vi "运维调试_CODMn.vi"() -> ()   [LabVIEW 2016, in "斯坦道CODMn新电路板.lvlib"]
uses:
  <vilib>/Utility/miscctls.llb/LVPointTypeDef.ctl
  <vilib>/Waveform/WDTFileIO.llb/Read Waveform from File.vi
  <vilib>/ptbypt/NI_PtbyPt.lvlib
panel:
  in  "告警代码":u16
  in  "周期设置":bool
  out "消解压力kPa":sgl format="%#.2f"
  out "权限等级":string
  out "总步数":i32
  out "滑动杆":u8(slide) caption="测试进度" scale=0.0..100.0
  in  "参数查询":bool
  in  "仪器校准":bool
  out "仪器版本号":string
  in  "试剂余量设置":bool
  out "试剂余量显示":sgl[][](graph)
  in  "公式切换阈值滴定数(0~9999)":dbl
  out "X0":u16
  in  "平台反控标样校准":enum16{"标液1", "标液2", "标液3"}(ring)
  in  "平台反控校准量程":enum16{"低量程1", "低量程2", "高量程1", "高量程2"}(ring)
  out "注射泵保温温度":sgl format="%#.2f"
  in  "历史波形 2":bool
  in  "返回 3":bool
  out "时间-温度":u16[](array[numeric]) caption="数组"
  out "温度波形时间":timestamp
  out "ORP滴定曲线 2":u16[](graph)
  in  "历史波形":bool
  in  "返回 2":bool
  out "滴定数-ORP值":u16[](array[numeric]) caption="数组"
  out "波形时间":timestamp
  out "ORP滴定曲线":u16[](graph)
  in  "滴定曲线":bool
  out "终点滴定数":sgl format="%#.2f"
  out "单位:":T1(ring)
  out "运行状态":T2 {"数据时间:" format="%<%y/%m/%d %H:%M:%S>T"; "仪器时间:" format="%<%y/%m/%d %H:%M:%S>T"}
  out "模块版本号":string
  out "当前步骤剩余时间":sgl format="%#.2f"
  out "加热实时温度":sgl format="%#.2f"
  out "ORP值/光值":sgl format="%#.2f"
  in  "布尔":bool
  in  "流程固件":bool
  in  "公式单个写入":bool
  in  "流程路径":path=path "C:/Users/STD/Documents/斯坦道流程文件/流程.xml"
  out "字符串":string
  out "运行时间":sgl format="%#.2f"
  out "环境湿度":sgl format="%#.2g"
  out "环境温度":sgl format="%#.2g"
  in  "数组":string[](array[string])
  in  "量程切换阈值写入":bool
  in  "量程切换阈值读取":bool
  in  "参数下拉列表":enum16{"CODMn"}(ring)
  in  "量程下拉列表":enum16{"低量程1", "低量程2", "高量程1", "高量程2"}(ring)
  in  "测量模式下拉列表":T3(ring)=enum."水样测量"
  in  "公式":cluster{"X^2":dbl, "X":dbl, "b":dbl}
  in  "写公式":bool
  in  "读公式":bool
  in  "返回":bool
  in  "设置":bool
  out "集成报警信息":string
  in  "停止":bool
  in  "手动启动":bool
  in  "单步测试":bool
  out "当前滴定数":sgl format="%#.2f"
  out "K":sgl format="%#.2f"
  out "B":sgl format="%#.2f"
  out "A":sgl format="%#.2f"
  out "多列列表框":i32(listbox)
  # "."
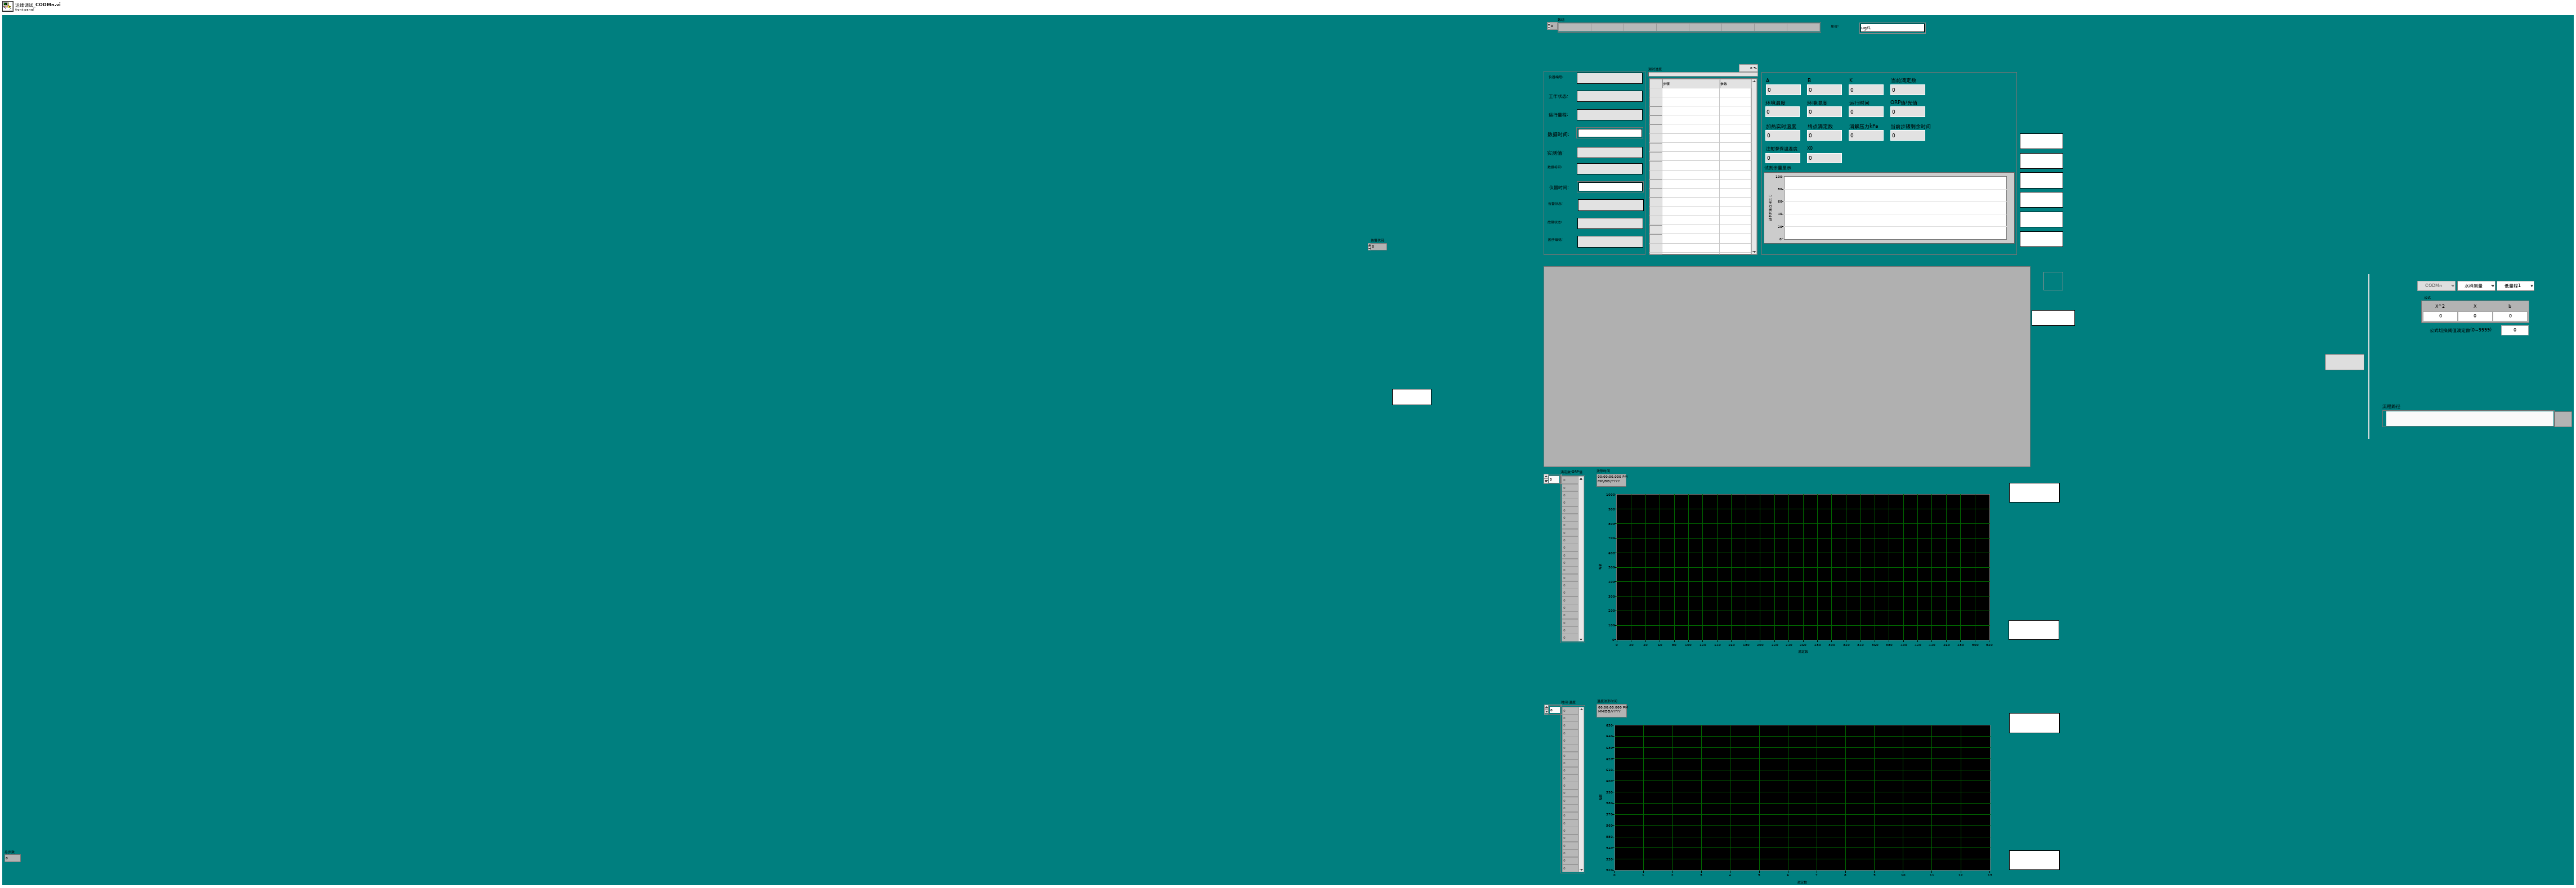
[diagram p1: front panel]
types:
  T1 = enum16{"ug/L", "mg/L", "ppm", "mg/m3", "cm", "ppb", "ug/m3", "%", "nmol/mol", "umol/mol", "MPN/L", "MPN/100ml", "ng/m3", "NTU", "无量纲", "ms/cm", "us/cm", "℃", "mV", "万个/L"}
  T2 = cluster{"仪器编号:":string, "工作状态:":string, "运行量程: ":string, "数据时间:":timestamp, "实测值:":string, "数据标识: ":string, "仪器时间:":timestamp, "告警状态: ":string, "故障状态:  ":string, "因子编码:":string}
  T3 = enum16{"", "水样测量", "标样核查", "零点核查", "跨度核查", "空白测试", "平行样测试", "加标回收"}
  T4 = cluster{"Major":u16, "Minor":u16, "Fix":u16, "Build":u16}
  T5 = cluster{"测量量程":sgl, "测量检出限":sgl, "测量精度":sgl, "测量间隔":sgl, "消解温度":sgl, "消解时长":sgl, "三项式系数":sgl, "二次多项式系数":sgl, "曲线斜率":sgl, "曲线截距":sgl, "线性相关系数":sgl, "空白校准时间":timestamp, "标样校准时间":timestamp, "测量信号值":sgl, "稀释倍数":sgl, "量程系数":sgl}
  T6 = typedef "LVPointTypeDef.ctl" = cluster{"Horizontal":i16, "Vertical":i16}
  T7 = cluster{"因子编码":u32, "单位":u16, "标样参考值":sgl, "水样数据时间":timestamp, "水样实测值":sgl, "水样数据标识":string, "标样数据时间":timestamp, "标样实测值":sgl, "标样数据标识":string, "空白数据时间":timestamp, "空白实测值":sgl, "空白数据标识":string, "零点核查数据时间":timestamp, "零点核查实测值":sgl, "零点核查数据标识":string, "跨度核查数据时间":timestamp, "跨度核查实测值":sgl, "跨度核查数据标识":string, "加标回收数据时间":timestamp, "加标回收实测值":sgl, "加标回收数据标识":string, "平行样数据时间":timestamp, "平行样实测值":sgl, "平行样数据标识":string, "F0":sgl, "F1":sgl, "F2":sgl, "F3":sgl, "F4":sgl, "F5":sgl, "F6":sgl, "F7":sgl, "温度":sgl, "湿度":sgl, "X值":sgl, "fidrange":u16}
  T8 = cluster{"系统时间":timestamp, "工作状态":u16, "测量模式":enum16{"待机", "连续模式", "周期模式", "定点模式", "受控模式", "手动模式"}, "告警代码":u16, "故障代码":u16, "日志代码":u16, "软件版本":u16, "A":sgl, "B":sgl, "K":sgl, "当前滴定数":sgl, "T":sgl, "H":sgl, "id":u16, "flowid":u16, "量程":u16, "加热实时温度":sgl, "当前ORP值":sgl, "运行时间":sgl, "当前步骤剩余时间":sgl, "结束滴定数":sgl, "注射泵保温温度":sgl, "匹配滴定数X0":u16, "X^2":sgl, "X":sgl, "B 2":sgl, "光值1":sgl, "光值2":sgl, "光值3":sgl, "光值4":sgl, "光值5":sgl, "光值6":sgl, "光值7":sgl, "光值8":sgl}
  T9 = typedef "Alarm interface.lvlib/报警短信语音交互.ctl" = cluster{"参数":string, "元器件":string, "故障现象":string, "code":string, "platform_alarm_code":string, "solutionList":cluster{"reason":string, "solution":string}[], "是否上报":string}
  T10 = enum8{"Enabled", "Disabled", "Disabled and Grayed Out"}
  T11 = enum16{"空闲", "水样测试", "标样核查", "零点核查", "跨度核查", "空白测试", "平行样测试", "加标回收", "空白校准", "标样校准", "初始化（清洗）"}
  T12 = typedef "TimingControl.lvlib/TimingControl.lvclass/国标控制命令.ctl" = enum16{"启动测量", "标样核查", "零点核查", "跨度核查", "空白测试", "平行样测试", "加标回收", "空白校准", "标样校准", "初始化（清洗）", "停止测试", "仪器重启", "校时", "模式设置", "测量间隔设置"}
  T13 = typedef "TimingControl.lvlib/TimingControl.lvclass/测量参数.ctl" = u16
  T14 = cluster{"时间标识":timestamp, "设备":string, "日志信息":string, "流程参数":string}
  T15 = typedef "LVRowAndColumnUnsignedTypeDef.ctl" = cluster{"Row":u32, "Column":u32}
  T16 = enum32{"Bad", "Idle", "Run top level", "Running"}
  T17 = cluster{"站号":u16, "量程切换":enum32{"H", "L", "AUTO"}, "控制命令":u16, "模式设置":enum16{"待机", "连续模式", "周期模式", "定点模式", "受控模式", "手动模式"}, "测量间隔":u16}
  T18 = cluster{"测量量程":dbl, "测量精度":dbl, "测量间隔":dbl, "消解温度":dbl, "消解时长":dbl, "空白校准时间":timestamp, "曲线截距":dbl, "曲线斜率":dbl, "测量检出限":dbl, "测量信号值":dbl, "线性相关系数":dbl, "二次多项式系数":dbl, "标样校准时间":timestamp, "稀释倍数":dbl, "三项式系数":dbl, "空白标定系数":dbl, "量程系数":dbl, "F0/ORPA":dbl, "F1/ORPB":dbl, "F2/ORPK":dbl, "F3":dbl, "F4":dbl, "F5":dbl, "F6":dbl, "F7":dbl, "X0/滴定数":dbl, "量程":dbl}
  T19 = cluster{"跨度值":dbl, "零点标准液浓度":dbl, "跨度标准液浓度":dbl, "标准液标准浓度":dbl, "零点标准液偏差":dbl, "跨度标准液偏差":dbl, "标准液标准偏差":dbl}
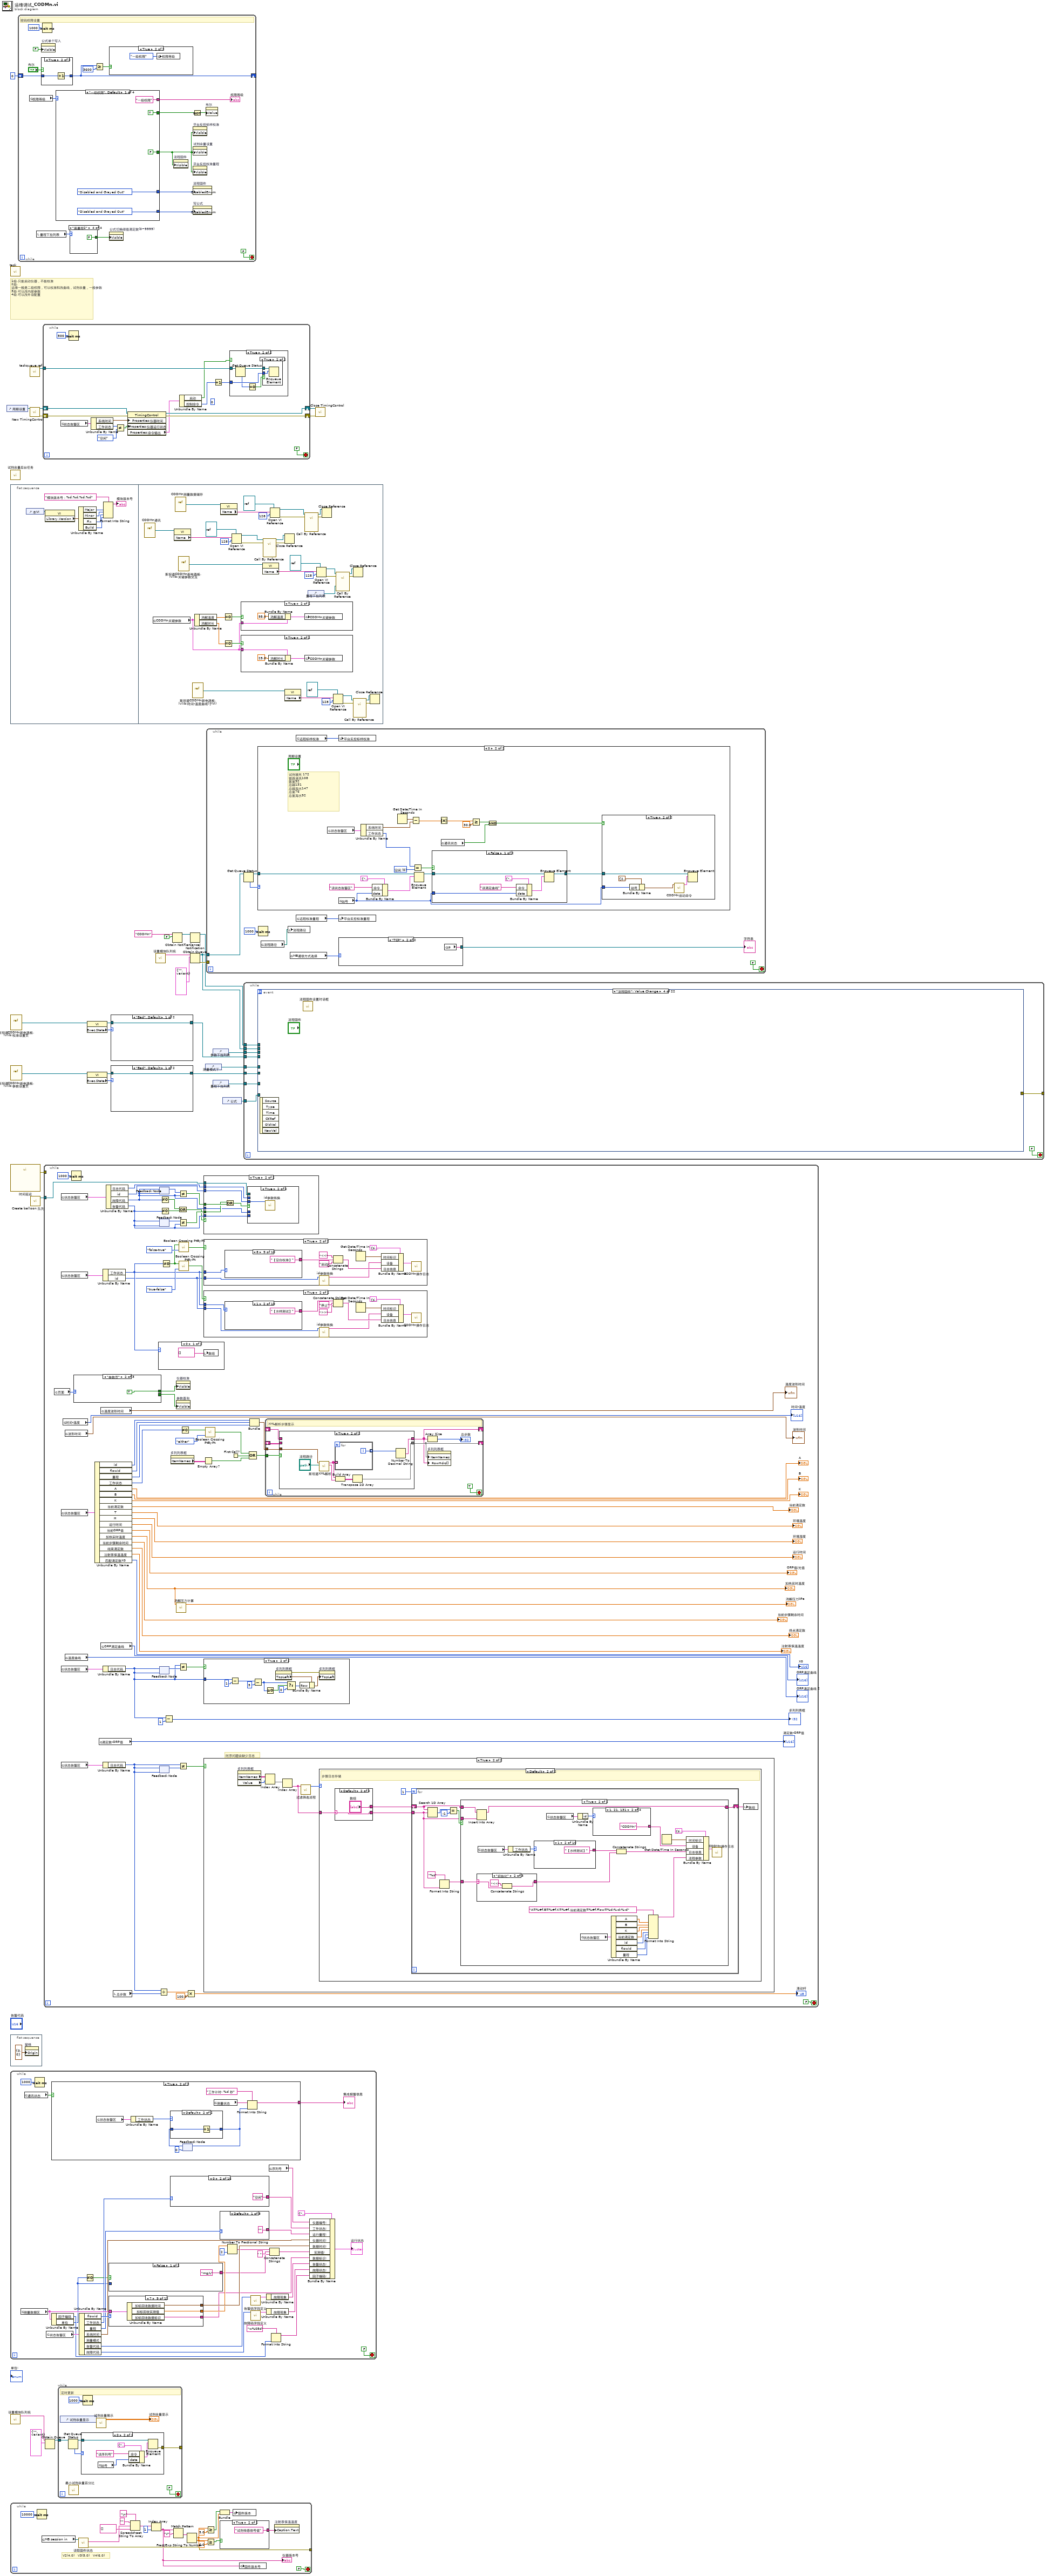
[diagram p0: block diagram]
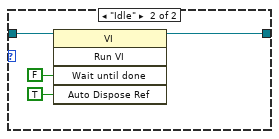
[diagram p2: hidden frame]
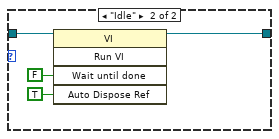
[diagram p3: hidden frame]
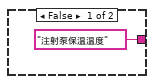
[diagram p4: hidden frame]
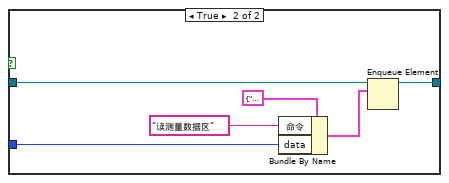
[diagram p7: hidden frame]
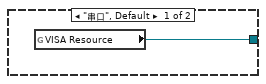
[diagram p9: hidden frame]
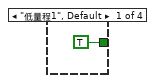
[diagram p12: hidden frame]
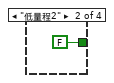
[diagram p13: hidden frame]
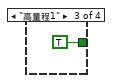
[diagram p14: hidden frame]
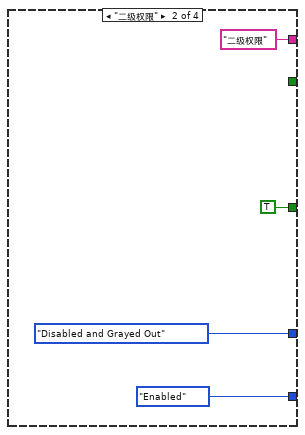
[diagram p15: hidden frame]
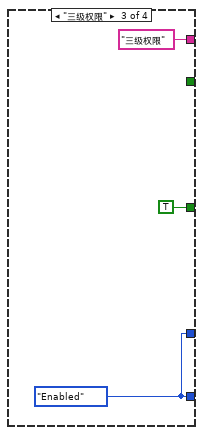
[diagram p16: hidden frame]
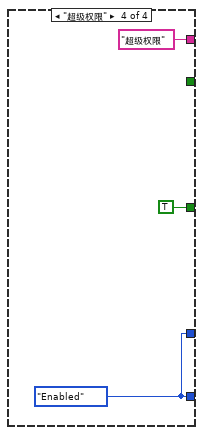
[diagram p17: hidden frame]
diagram:
  # "1级.只能启动仪器，不能校准\n2级.运维一般是二级权限，可以校准和改曲线，试剂余量，一般参数\n3级.可以改内部参数\n4级.可以改外设配置"
  n1 = control-ref of="周期设置"() -> (w5:refnum<vi>)
  n2 = call "task.vi"() -> ()  [unwired: 12 in]
  n3 = call "试剂余量后台任务.vi"() -> ()  [unwired: 12 in]
  n4 = flat-sequence {
    frame #0 {
      n5 = control-ref of="本VI"() -> (w40:refnum<vi>)
      n6 = property class="VI"(reference=w40) -> ("Library.Version"=w39:T4)  [unwired: 1 in, 2 out]
      n7 = Unbundle By Name(w39) -> ("Major"=w37:u16, "Minor"=w36:u16, "Fix"=w35:u16, "Build"=w34:u16)
      n8 = Format Into String(format string="模块版本号：%d.%d.%d.%d" ("格式字符串"), w37, w36, w35, w34) -> (resulting string=→"模块版本号":string)  [unwired: 2 in, 1 out]
    }
    frame #1 {
      n9 = vi-ref "CODMn通讯.vi"() -> (w54:refnum<vi>)
      n10 = global read "CODMn断电保存全局变量.vi" "CODMn关键参数"() -> (w41:T5)
      n11 = property class="VI"(reference=w54) -> ("Name"=w53:string)  [unwired: 1 in, 2 out]
      n12 = vi-ref "CODMn测量数据储存.vi"() -> (w78:refnum<vi>)
      n13 = vi-ref "斯坦道CODMn新电路板.lvlib:关键参数交互.vi"() -> (w64:refnum<vi>)
      n14 = vi-ref "斯坦道CODMn新电路板.lvlib:时间-温度曲线(子VI).vi"() -> (w56:refnum<vi>)
      n15 = Unbundle By Name(w41) -> ("消解温度"=w45:sgl, "消解时长"=w42:sgl)
      n16 = property class="VI"(reference=w78) -> ("Name"=w71:string)  [unwired: 1 in, 2 out]
      n17 = Equal To 0?(x=w45) -> (x = 0?=w44:bool)
      n18 = Equal To 0?(x=w42) -> (x = 0?=w43:bool)
      n19 = Open VI Reference(type specifier VI Refnum (for type only)=refnum<vi> refnum, vi path=w53, options=128 ("选项")) -> (vi reference=w51:refnum<vi>, error out=w49:errorcluster)  [unwired: 3 in]
      n20 = case shown="True" w44 {
        tunnel: w41 -> [_ w84]
        frame False {
        }
        frame True {
          n21 = Bundle By Name(cluster=w84, "消解温度"=sgl 95.0) -> (w83:T5)
          n22 = global write "CODMn断电保存全局变量.vi" "CODMn关键参数"(w83) -> ()
        }
      }
      n23 = case shown="True" w43 {
        tunnel: w41 -> [_ w81]
        frame False {
        }
        frame True {
          n24 = Bundle By Name(cluster=w81, "消解时长"=sgl 25.0) -> (w80:T5)
          n25 = global write "CODMn断电保存全局变量.vi" "CODMn关键参数"(w80) -> ()
        }
      }
      n26 = property class="VI"(reference=w64) -> ("Name"=w70:string)  [unwired: 1 in, 2 out]
      n27 = call-by-ref "?"(reference=w51, error in=w49) -> (reference out=w47:refnum<vi>, error out=w48:errorcluster)  [unwired: 12 in]
      n28 = Open VI Reference(type specifier VI Refnum (for type only)=refnum<vi> refnum, vi path=w71, options=128 ("选项")) -> (vi reference=w73:refnum<vi>, error out=w75:errorcluster)  [unwired: 3 in]
      n29 = Close Reference(reference=w47, error in (no error)=w48) -> ()  [unwired: 1 out]
      n30 = property class="VI"(reference=w56) -> ("Name"=w62:string)  [unwired: 1 in, 2 out]
      n31 = call-by-ref "?"(reference=w73, error in=w75) -> (reference out=w77:refnum<vi>, error out=w76:errorcluster)  [unwired: 12 in]
      n32 = control-ref of="量程下拉列表"() -> (w46:refnum<vi>)
      n33 = Open VI Reference(type specifier VI Refnum (for type only)=refnum<vi> refnum, vi path=w70, options=128 ("选项")) -> (vi reference=w68:refnum<vi>, error out=w67:errorcluster)  [unwired: 3 in]
      n34 = Close Reference(reference=w77, error in (no error)=w76) -> ()  [unwired: 1 out]
      n35 = Open VI Reference(type specifier VI Refnum (for type only)=refnum<vi> refnum, vi path=w62, options=128 ("选项")) -> (vi reference=w60:refnum<vi>, error out=w59:errorcluster)  [unwired: 3 in]
      n36 = call-by-ref "?"(reference=w68, error in=w67, "量程下拉列表"=w46) -> (reference out=w65:refnum<vi>, error out=w66:errorcluster)  [unwired: 11 in]
      n37 = Close Reference(reference=w65, error in (no error)=w66) -> ()  [unwired: 1 out]
      n38 = call-by-ref "?"(reference=w60, error in=w59) -> (reference out=w57:refnum<vi>, error out=w58:errorcluster)  [unwired: 12 in]
      n39 = Close Reference(reference=w57, error in (no error)=w58) -> ()  [unwired: 1 out]
    }
  }
  n40 = vi-ref "斯坦道CODMn新电路板.lvlib:校准设置页.vi"() -> (w16:refnum<vi>)
  n41 = vi-ref "斯坦道CODMn新电路板.lvlib:参数设置页.vi"() -> (w13:refnum<vi>)
  n42 = call "时间延迟"() -> ("error out"=w26:errorcluster)  [unwired: 11 in]
  n43 = flat-sequence {
    frame #0 {
      n44 = property on="窗格" class="Pane"("Origin"=T6 {"Horizontal"=0, "Vertical"=0} ("原点")) -> ()  [unwired: 2 in, 2 out]
    }
  }
  n45 = while {
    stop <- FALSE stop-if-true
    n46 = global read "VARCODMn全局变量.vi" "测量数据区"() -> (w113:T7)
    n47 = global read "VARCODMn全局变量.vi" "通讯状态"() -> (w117:bool)
    n48 = Wait (ms)(milliseconds to wait=u32 1000 ("等待时间（毫秒）")) -> ()  [unwired: 1 out]
    n49 = global read "VARCODMn全局变量.vi" "状态告警区"() -> (w115:T8)
    n50 = case shown="True" w117 {
      tunnel: ["通讯异常" ("集成报警信息") w195] -> w116
      frame False {
      }
      frame True {
        n51 = global read "VARCODMn全局变量.vi" "状态告警区"() -> (w201:T8)
        n52 = Unbundle By Name(w201) -> ("工作状态"=w200:u16)
        n53 = feedback #1(0) -> (w198:i32)
        n54 = case shown="Default" w200 {
          tunnel: w198 -> [_ w203]
          tunnel: [_ w202] -> w196
          frame 0 {
          }
          frame Default {
            n55 = Increment(x=w203) -> (x+1=w202:i32)
          }
        }
        n56 = feedback-in #1(w196) -> ()
        n57 = global read "VARCODMn全局变量.vi" "测量状态"() -> (w194:string)
        n58 = Format Into String(format string="工作计时: %d 秒" ("格式字符串"), initial string=w194, w196) -> (resulting string=w195:string)  [unwired: 1 in, 1 out]
      }
    }
    "集成报警信息" <- w116
    n59 = Unbundle By Name(w113) -> ("因子编码"=w93:u32, "单位"=w90:u16)
    n60 = Unbundle By Name(w115) -> ("flowid"=w114:u16, "工作状态"=w111:u16, "量程"=w109:u16, "系统时间"=w107:timestamp, "告警代码"=w97:u16, "故障代码"=w96:u16)  [unwired: 1 out]
    n61 = Not Equal To 0?(x=w90) -> (x != 0?=w91:bool)
    n62 = case shown="False" w91 {
      tunnel: ["mg/L" ("RingText.Text") w122] -> w95
      tunnel: w90 -> [_ w121]
      frame False {
      }
      frame True {
        n63 = property on="单位:" class="Enum (strict)"("Value"=w121) -> (error out=w123:errorcluster)  [unwired: 2 in, 1 out]
        n64 = property on="单位:" class="Enum (strict)"(error in=w123) -> ("RingText.Text"=w122:string)  [unwired: 1 in, 2 out]
      }
    }
    n65 = case shown="7" w114 {
      selector: w114 -> [w146 _ _ _ _ _ _ _ _ _ _ _]
      tunnel: [_ w152 w156 w160 w164 w168 w172 w176 w180 w183 w187 w192] -> w104
      tunnel: [_ w150 w155 w159 w163 w167 w171 w174 w179 w182 w186 w191] -> w99
      tunnel: [_ w149 w154 w158 w162 w166 w170 w173 w178 w181 w185 w190] -> w98
      tunnel: w113 -> [_ w151 w153 w157 w161 w165 w169 w175 w177 w184 w188 w189]
      frame Default {
        n66 = Format Into String(format string="%d" ("格式字符串"), initial string="未知" ("工作状态"), w146) -> ()  [unwired: 1 in, 2 out]
      }
      frame 0 {
        n67 = Unbundle By Name(w151) -> ("水样数据时间"=w152:timestamp, "水样实测值"=w150:sgl, "水样数据标识"=w149:string)
      }
      frame 1 {
        n68 = Unbundle By Name(w153) -> ("水样数据时间"=w156:timestamp, "水样实测值"=w155:sgl, "水样数据标识"=w154:string)
      }
      frame 2 {
        n69 = Unbundle By Name(w157) -> ("标样数据时间"=w160:timestamp, "标样实测值"=w159:sgl, "标样数据标识"=w158:string)
      }
      frame 3 {
        n70 = Unbundle By Name(w161) -> ("零点核查数据时间"=w164:timestamp, "零点核查实测值"=w163:sgl, "零点核查数据标识"=w162:string)
      }
      frame 4 {
        n71 = Unbundle By Name(w165) -> ("跨度核查数据时间"=w168:timestamp, "跨度核查实测值"=w167:sgl, "跨度核查数据标识"=w166:string)
      }
      frame 5 {
        n72 = Unbundle By Name(w169) -> ("空白数据时间"=w172:timestamp, "空白实测值"=w171:sgl, "空白数据标识"=w170:string)
      }
      frame 6 {
        n73 = Unbundle By Name(w175) -> ("平行样数据时间"=w176:timestamp, "平行样实测值"=w174:sgl, "平行样数据标识"=w173:string)
      }
      frame 7 {
        n74 = Unbundle By Name(w177) -> ("加标回收数据时间"=w180:timestamp, "加标回收实测值"=w179:sgl, "加标回收数据标识"=w178:string)
      }
      frame 8 {
        n75 = Unbundle By Name(w184) -> ("空白数据时间"=w183:timestamp, "空白实测值"=w182:sgl, "空白数据标识"=w181:string)
      }
      frame 9 {
        n76 = Unbundle By Name(w188) -> ("标样数据时间"=w187:timestamp, "标样实测值"=w186:sgl, "标样数据标识"=w185:string)
      }
      frame 10 {
        n77 = Unbundle By Name(w189) -> ("水样数据时间"=w192:timestamp, "水样实测值"=w191:sgl, "水样数据标识"=w190:string)
      }
    }
    n78 = case shown="0" w111 {
      selector: w111 -> [w127 _ _ _ _ _ _ _ _ _ _ _ _ _ _ _]
      tunnel: [w128 "空闲" ("工作状态") "水样测量" ("工作状态") "标样核查" ("工作状态") "零点核查" ("工作状态") "跨度核查" ("工作状态") "空白测试" ("工作状态") "平行样测试" ("工作状态") "加标回收" ("工作状态") "空白校准" ("工作状态") "标样校准" ("工作状态") "初始化" ("工作状态") "调试" ("工作状态") "填充管路" ("工作状态") "清洗管路" ("工作状态") "清洗反应杯" ("工作状态")] -> w110
      frame Default {
        n79 = Format Into String(format string="%d" ("格式字符串"), initial string="未知" ("工作状态"), w127) -> (resulting string=w128:string)  [unwired: 1 in, 1 out]
      }
      frame 0 {
      }
      frame 1 {
      }
      frame 2 {
      }
      frame 3 {
      }
      frame 4 {
      }
      frame 5 {
      }
      frame 6 {
      }
      frame 7 {
      }
      frame 8 {
      }
      frame 9 {
      }
      frame 10 {
      }
      frame 22 {
      }
      frame 30 {
      }
      frame 31 {
      }
      frame 32 {
      }
    }
    n80 = case shown="Default" w109 {
      tunnel: ["" ("字符串") "低量程" ("字符串") "高量程" ("字符串")] -> w108
      frame Default {
      }
      frame 0 {
      }
      frame 1 {
      }
    }
    n81 = Number To Fractional String(number=w99, precision (6)=i16 2 ("精度(6)")) -> (F-format string=w102:string)  [unwired: 2 in]
    n82 = call "告警码字段定义.vi"("告警代码"=w97) -> ("data"=w89:T9)  [unwired: 10 in]
    n83 = call "故障码字段定义.vi"("故障代码"=w96) -> ("data"=w88:T9)  [unwired: 10 in]
    n84 = Unbundle By Name(w89) -> ("故障现象"=w86:string)
    n85 = Unbundle By Name(w88) -> ("故障现象"=w87:string)
    n86 = global read "VARCODMn全局变量.vi" "序列号"() -> (w112:string)
    n87 = Concatenate Strings(w102, " " ("字符串"), w95) -> (w100:string)
    n88 = Format Into String(format string="w%05d" ("格式字符串"), w93) -> (resulting string=w92:string)  [unwired: 2 in, 1 out]
    n89 = Bundle By Name(cluster=T2 {"仪器编号:"="", "工作状态:"="", "运行量程: "="", "数据时间:"=timestamp(0 s since 1904-01-01), "实测值:"="", "数据标识: "="", "仪器时间:"=timestamp(0 s since 1904-01-01), "告警状态: "="", "故障状态:  "="", "因子编码:"=""} ("运行状态"), "仪器编号:"=w112, "工作状态:"=w110, "运行量程:"=w108, "仪器时间:"=w107, "数据时间:"=w104, "实测值:"=w100, "数据标识:"=w98, "告警状态:"=w86, "故障状态:"=w87, "因子编码:"=w92) -> (→"运行状态":T2)
  }
  n90 = call "设置模块队列名.vi"() -> ("Msg"=w6:string)  [unwired: 11 in]
  n91 = while {
    tunnel: [w220] -> _
    stop <- FALSE stop-if-true
    # "V2(4.0)   V3(5.0)   V4(6.0)"
    n92 = Wait (ms)(milliseconds to wait=u32 10000 ("等待时间（毫秒）")) -> ()  [unwired: 1 out]
    n93 = global read "VARCODMn全局变量.vi" "MB session in"() -> (w221:refnum<class "MB_Master.lvclass">)
    n94 = call "读取固件状态.vi"("MB session in"=w221) -> ("error out"=w220:errorcluster, "结果字符串"=w216:string)  [unwired: 8 in, 1 out]
    n95 = Spreadsheet String To Array(delimiter (Tab)="\n" ("分隔符(Tab)"), format string="" ("格式字符串"), spreadsheet string=w216, array type (2D Dbl)=string[] []) -> (array=w215:string[])
    n96 = Index Array(array=w215, index=1 ("索引")) -> (element=w204:string)
    "仪器版本号" <- w204
    n97 = Match Pattern(string=w204, regular expression="V" ("正则表达式")) -> (after substring=w212:string)  [unwired: 1 in, 3 out]
    n98 = Fract/Exp String To Number(string=w212) -> (number=w206:dbl)  [unwired: 3 in, 1 out]
    n99 = Greater Or Equal?(x=w206, y=5.0) -> (x >= y?=w207:bool)
    n100 = Greater Or Equal?(x=w206, y=6.0) -> (x >= y?=w209:bool)
    n101 = Bundle(w207, w206) -> (w205:cluster{bool, dbl})  [unwired: 1 in]
    n102 = case shown="True" w209 {
      tunnel: ["注射泵保温温度" "试剂传感信号值"] -> w208
      frame False {
      }
      frame True {
      }
    }
    n103 = global write "VARCODMn全局变量.vi" "固件版本"(w205) -> ()
    n104 = global write "VARCODMn全局变量.vi" "固件版本号"(w204) -> ()
    n105 = property on="注射泵保温温度" class="DigNum (strict)"("Caption.Text"=w208) -> ()  [unwired: 2 in, 2 out]
  }
  n106 = while {
    shift-right: [w239] -> _
    shift-left: u32 0 ("等待时间（毫秒）") -> [w240]
    stop <- FALSE stop-if-true
    # "密码权限设置"
    n107 = global read "VARCODMn全局变量.vi" "权限等级"() -> (w231:enum16{"一级权限", "二级权限", "三级权限", "超级权限"})
    n108 = local read "量程下拉列表"() -> (w233:enum16{"低量程1", "低量程2", "高量程1", "高量程2"})
    n109 = property on="公式单个写入" class="Bool"("Visible"=FALSE ("可见")) -> ()  [unwired: 2 in, 2 out]
    n110 = case shown="True" "布尔" {
      tunnel: w240 -> [_ w264]
      tunnel: [_ w263] -> w239
      frame False {
      }
      frame True {
        n111 = Increment(x=w264) -> (x+1=w263:u32)
      }
    }
    n112 = Wait (ms)(milliseconds to wait=u32 1000 ("等待时间（毫秒）")) -> ()  [unwired: 1 out]
    n113 = case shown="\"一级权限\", Default" w231 {
      tunnel: [T10."Disabled and Grayed Out" ("f") T10."Enabled" ("禁用") w258 w261] -> w234
      tunnel: [T10."Disabled and Grayed Out" ("f") T10."Disabled and Grayed Out" ("f") w258 w261] -> w235
      tunnel: [FALSE ("可见") TRUE ("可见") TRUE ("可见") TRUE ("可见")] -> w230
      tunnel: ["一级权限" "二级权限" "三级权限" "超级权限"] -> w229
      tunnel: [TRUE _ _ _] -> w228
      frame "一级权限", Default {
      }
      frame "二级权限" {
      }
      frame "三级权限" {
        w258 = T10."Enabled" ("禁用")
      }
      frame "超级权限" {
        w261 = T10."Enabled" ("禁用")
      }
    }
    "权限等级" <- w229
    n114 = case shown="\"高量程2\"" w233 {
      tunnel: [TRUE ("可见") FALSE ("可见") TRUE ("可见") FALSE ("可见")] -> w232
      frame "低量程1", Default {
      }
      frame "低量程2" {
      }
      frame "高量程1" {
      }
      frame "高量程2" {
      }
    }
    n115 = Greater Or Equal?(x=w239, y=u32 3600) -> (x >= y?=w237:bool)
    n116 = case shown="True" w237 {
      frame False {
      }
      frame True {
        n117 = global write "VARCODMn全局变量.vi" "权限等级"(enum16{"一级权限", "二级权限", "三级权限", "超级权限"}."一级权限" ("权限等级")) -> ()
      }
    }
    n118 = property on="公式切换阈值滴定数(0~9999)" class="DigNum (strict)"("Visible"=w232) -> ()  [unwired: 2 in, 2 out]
    n119 = property on="流程固件" class="Bool"("Visible"=w230) -> ()  [unwired: 2 in, 2 out]
    n120 = Not(x=w228) -> (.not. x?=w226:bool)
    n121 = property on="平台反控标样校准" class="Enum (strict)"("Visible"=w230) -> ()  [unwired: 2 in, 2 out]
    n122 = property on="试剂余量设置" class="Bool"("Visible"=w230) -> ()  [unwired: 2 in, 2 out]
    n123 = property on="平台反控校准量程" class="Enum (strict)"("Visible"=w230) -> ()  [unwired: 2 in, 2 out]
    n124 = property on="流程固件" class="Bool"("DisabledEnum"=w235) -> ()  [unwired: 2 in, 2 out]
    n125 = property on="写公式" class="Bool"("DisabledEnum"=w234) -> ()  [unwired: 2 in, 2 out]
    n126 = property on="布尔" class="Bool (strict)"("Value"=w226) -> ()  [unwired: 2 in, 2 out]
  }
  n127 = call "taskqueue ref.vi"() -> ("队列输出"=w8:refnum<queue>)  [unwired: 10 in, 1 out]
  n128 = call "New TimingControl.vi"("Reference"=w5) -> ("error out"=w3:errorcluster, "TimingControl out"=w4:refnum<class "TimingControl.lvclass">)  [unwired: 9 in]
  n129 = call "Create balloon 队列.vi"() -> ("队列输出"=w19:refnum<queue>)  [unwired: 11 in]
  n130 = while {
    tunnel: w8 -> [w276]
    shift-right: [w272] -> w2
    shift-left: w4 -> [w274]
    shift-right: [w271] -> w1
    shift-left: w3 -> [w273]
    stop <- FALSE stop-if-true
    (unwired) u32 0 ("f")
    n131 = global read "VARCODMn全局变量.vi" "状态告警区"() -> (w278:T8)
    n132 = Wait (ms)(milliseconds to wait=u32 500 ("等待时间（毫秒）")) -> ()  [unwired: 1 out]
    n133 = Unbundle By Name(w278) -> ("系统时间"=w269:timestamp, "工作状态"=w275:u16)
    n134 = Not Equal?(x=w275, y=T11."空闲") -> (x != y?=w268:bool)
    n135 = property class="TimingControl"(reference=w274, error in=w273, "Properties:仪器时间"=w269, "Properties:仪器运行状态"=w268) -> (reference out=w272:refnum<class "TimingControl.lvclass">, error out=w271:errorcluster, "Properties:命令输出"=w270:cluster{"启动":bool, "控制命令":T12, "测量参数":T13})
    n136 = Unbundle By Name(w270) -> ("启动"=w265:bool, "控制命令"=w267:T12)
    n137 = Increment(x=w267) -> (x+1=w266:T12)
    n138 = case shown="True" w265 {
      tunnel: w276 -> [_ w285]
      tunnel: w266 -> [_ w284]
      frame False {
      }
      frame True {
        n139 = Get Queue Status(queue=w285) -> (queue out=w283:refnum<queue>, # elements in queue=w282:i32)  [unwired: 2 in, 6 out]
        n140 = Equal To 0?(x=w282) -> (x = 0?=w281:bool)
        n141 = case shown="True" w281 {
          tunnel: w284 -> [_ w287]
          tunnel: w283 -> [_ w286]
          frame False {
          }
          frame True {
            n142 = Enqueue Element(queue=w286, element=w287) -> ()  [unwired: 2 in, 3 out]
          }
        }
      }
    }
  }
  n143 = while {
    tunnel: w26 -> [_]
    tunnel: w19 -> [w316]
    stop <- FALSE stop-if-true
    # "时序问题会缺少日志"
    n144 = global read "VARCODMn全局变量.vi" "页面"() -> (w293:enum16{"主页", "参数页", "校准页"})
    n145 = global read "VARCODMn全局变量.vi" "状态告警区"() -> (w344:T8)
    n146 = global read "VARCODMn全局变量.vi" "状态告警区"() -> (w340:T8)
    n147 = global read "VARCODMn全局变量.vi" "状态告警区"() -> (w353:T8)
    n148 = global read "VARCODMn全局变量.vi" "状态告警区"() -> (w319:T8)
    n149 = global read "VARCODMn全局变量.vi" "状态告警区"() -> (w338:T8)
    n150 = global read "VARCODMn全局变量.vi" "时间-温度"() -> (→"时间-温度":u16[])
    n151 = global read "VARCODMn全局变量.vi" "波形时间"() -> (→"波形时间":timestamp)
    n152 = global read "VARCODMn全局变量.vi" "温度曲线"() -> (→"ORP滴定曲线 2":u16[])
    n153 = Wait (ms)(milliseconds to wait=u32 1000 ("等待时间（毫秒）")) -> ()  [unwired: 1 out]
    n154 = case shown="\"参数页\"" w293 {
      tunnel: [_ _ TRUE ("可见")] -> w292
      tunnel: [_ TRUE ("可见") _] -> w291
      frame "主页", Default {
      }
      frame "参数页" {
      }
      frame "校准页" {
      }
    }
    n155 = Unbundle By Name(w353) -> ("id"=w350:u16, "flowid"=w352:u16, "量程"=w351:u16, "工作状态"=w330:u16, "A"=→"A":sgl, "B"=→"B":sgl, "K"=→"K":sgl, "当前滴定数"=→"当前滴定数":sgl, "T"=→"环境温度":sgl, "H"=→"环境湿度":sgl, "运行时间"=→"运行时间":sgl, "当前ORP值"=→"ORP值/光值":sgl, "加热实时温度"=w290:sgl, "当前步骤剩余时间"=→"当前步骤剩余时间":sgl, "结束滴定数"=→"终点滴定数":sgl, "注射泵保温温度"=→"注射泵保温温度":sgl, "匹配滴定数X0"=→"X0":u16)
    "加热实时温度" <- w290
    n156 = global read "VARCODMn全局变量.vi" "滴定数-ORP值"() -> (→"滴定数-ORP值":u16[])
    n157 = global read "VARCODMn全局变量.vi" "温度波形时间"() -> (→"温度波形时间":timestamp)
    n158 = global read "VARCODMn全局变量.vi" "ORP滴定曲线"() -> (→"ORP滴定曲线":u16[])
    n159 = Unbundle By Name(w340) -> ("工作状态"=w323:u16, "id"=w322:u16)
    n160 = Unbundle By Name(w319) -> ("日志代码"=w335:u16)
    n161 = Unbundle By Name(w338) -> ("日志代码"=w296:u16)
    n162 = Unbundle By Name(w344) -> ("日志代码"=w288:u16, "id"=w343:u16, "故障代码"=w302:u16, "告警代码"=w301:u16)
    n163 = local read "总步数"() -> (w295:i32)
    n164 = case shown="0" w323 {
      frame 0 {
        n165 = local write "数组"(string[] [] ("数组")) -> ()
      }
      frame 1, Default {
      }
    }
    n166 = Divide(x=w296, y=w295) -> (x/y=w298:dbl)
    n167 = feedback #2(w302) -> (w341:u16)
    n168 = feedback-in #2(w302) -> ()
    n169 = feedback #3(w301) -> (w318:u16)
    n170 = feedback-in #3(w301) -> ()
    n171 = feedback-in #4(w335) -> ()
    n172 = feedback #4(w335) -> (w358:u16)
    n173 = feedback #5(w296) -> (w339:u16)
    n174 = feedback-in #5(w296) -> ()
    n175 = Not Equal To 0?(x=w302) -> (x != 0?=w304:bool)
    n176 = Not Equal To 0?(x=w301) -> (x != 0?=w303:bool)
    n177 = Not Equal To 0?(x=w323) -> (x != 0?=w325:bool)
    n178 = Subtract(x=w335, y=1) -> (x-y=→"多列列表框":i32)
    n179 = property on="多列列表框" class="MCListbox (strict)"() -> ("ItemNames"=w314:string[][])  [unwired: 2 in, 2 out]
    n180 = property on="仪器校准" class="Bool"("Visible"=w291) -> ()  [unwired: 2 in, 2 out]
    n181 = property on="参数查询" class="Bool"("Visible"=w292) -> ()  [unwired: 2 in, 2 out]
    n182 = call "消解压力计算.vi"("当前消解温度"=w290) -> ("消解压力"=→"消解压力kPa":dbl)  [unwired: 10 in]
    n183 = Or(x=w304, y=w303) -> (x .or. y?=w300:bool)
    n184 = Not Equal?(x=w341, y=w302) -> (x != y?=w342:bool)
    n185 = Not Equal?(x=w318, y=w301) -> (x != y?=w317:bool)
    n186 = Not Equal?(x=w335, y=w358) -> (x != y?=w357:bool)
    n187 = Not Equal?(x=w296, y=w339) -> (x != y?=w337:bool)
    n188 = call <vilib>:"Boolean Crossing PtByPt.vi"("direction"=enum16{"either", "false-true", "true-false"}."false-true", "input"=w325) -> ("crossing"=w327:bool)  [unwired: 1 in]
    n189 = call <vilib>:"Boolean Crossing PtByPt.vi"("direction"=enum16{"either", "false-true", "true-false"}."true-false", "input"=w325) -> ("crossing"=w324:bool)  [unwired: 1 in]
    n190 = Not Equal To 0?(x=w330) -> (x != 0?=w355:bool)
    n191 = Multiply(x=w298, y=100.0) -> (x*y=→"滑动杆":dbl)
    n192 = case shown="True" w300 {
      tunnel: w343 -> [_ w476]
      tunnel: w342 -> [_ w475]
      tunnel: w317 -> [_ w473]
      tunnel: w301 -> [_ w472]
      tunnel: w316 -> [_ w471]
      tunnel: w302 -> [_ w470]
      tunnel: w288 -> [_ w469]
      frame False {
      }
      frame True {
        n193 = Or(x=w473, y=w475) -> (x .or. y?=w474:bool)
        n194 = case shown="True" w474 {
          tunnel: w476 -> [_ w477]
          tunnel: w470 -> [_ _]
          tunnel: w472 -> [_ _]
          tunnel: w471 -> [_ _]
          tunnel: w469 -> [_ _]
          frame False {
          }
          frame True {
            n195 = call "id参数转换.vi"("id"=w477) -> ()  [unwired: 10 in, 1 out]
          }
        }
      }
    }
    n196 = case shown="True" w327 {
      tunnel: w322 -> [_ w383]
      tunnel: w323 -> [_ w388]
      frame False {
      }
      frame True {
        n197 = case shown="8" w388 {
          tunnel: [_ "【水样测试】" ("字符串") "【标样核查】" ("字符串") "【零点核查】" ("字符串") "【跨度核查】" ("字符串") "【空白测试】" ("字符串") "【平行样测试】" ("字符串") "【加标回收】" ("字符串") "【空白校准】" ("字符串") "【标样校准】" ("字符串")] -> w387
          frame 0, Default {
          }
          frame 1 {
          }
          frame 2 {
          }
          frame 3 {
          }
          frame 4 {
          }
          frame 5 {
          }
          frame 6 {
          }
          frame 7 {
          }
          frame 8 {
          }
          frame 9 {
          }
        }
        n198 = call "id参数转换.vi"("id"=w383) -> ("table输出"=w382:string)  [unwired: 10 in]
        n199 = Concatenate Strings("<<" ("字符串"), w387, "启动" ("字符串")) -> (w386:string)
        n200 = Get Date/Time In Seconds() -> (seconds since 1Jan1904=w390:timestamp)
        n201 = Bundle By Name(cluster=T14 {"时间标识"=timestamp(0 s since 1904-01-01), "设备"="", "日志信息"="", "流程参数"=""} ("data in"), "时间标识"=w390, "设备"=w382, "日志信息"=w386) -> (w389:T14)
        n202 = call "CODMn操作日志.vi"("data in"=w389) -> ()  [unwired: 11 in]
      }
    }
    n203 = case shown="True" w324 {
      tunnel: w322 -> [_ w365]
      tunnel: w323 -> [_ w369]
      frame False {
      }
      frame True {
        n204 = case shown="1" w369 {
          tunnel: [_ "【水样测试】" ("字符串") "【标样核查】" ("字符串") "【零点核查】" ("字符串") "【跨度核查】" ("字符串") "【空白测试】" ("字符串") "【平行样测试】" ("字符串") "【加标回收】" ("字符串") "【空白校准】" ("字符串") "【标样校准】" ("字符串")] -> w368
          frame 0, Default {
          }
          frame 1 {
          }
          frame 2 {
          }
          frame 3 {
          }
          frame 4 {
          }
          frame 5 {
          }
          frame 6 {
          }
          frame 7 {
          }
          frame 8 {
          }
          frame 9 {
          }
        }
        n205 = call "id参数转换.vi"("id"=w365) -> ("table输出"=w364:string)  [unwired: 10 in]
        n206 = Concatenate Strings(w368, "停止" ("字符串"), ">>" ("字符串")) -> (w367:string)
        n207 = Get Date/Time In Seconds() -> (seconds since 1Jan1904=w371:timestamp)
        n208 = Bundle By Name(cluster=T14 {"时间标识"=timestamp(0 s since 1904-01-01), "设备"="", "日志信息"="", "流程参数"=""} ("data in"), "时间标识"=w371, "设备"=w364, "日志信息"=w367) -> (w370:T14)
        n209 = call "CODMn操作日志.vi"("data in"=w370) -> ()  [unwired: 11 in]
      }
    }
    n210 = Empty Array?(array=w314) -> (empty?=w313:bool)
    n211 = case shown="True" w357 {
      tunnel: w335 -> [_ w499]
      frame False {
      }
      frame True {
        n212 = Subtract(x=w499, y=1) -> (x-y=w497:i32)
        n213 = Subtract(x=w497, y=5) -> (x-y=w501:i32)
        n214 = Greater Or Equal To 0?(x=w501) -> (x >= 0?=w500:bool)
        n215 = property on="多列列表框" class="MCListbox (strict)"() -> (error out=w505:errorcluster, "TopLeft"=w506:T15)  [unwired: 2 in, 1 out]
        n216 = Select(t=w501, s=w500, f=0) -> (s? t:f=w502:i32)
        n217 = Bundle By Name(cluster=w506, "Row"=w502) -> (w507:T15)
        n218 = property on="多列列表框" class="MCListbox (strict)"(error in=w505, "TopLeft"=w507) -> ()  [unwired: 1 in, 2 out]
      }
    }
    n219 = case shown="True" w337 {
      frame False {
      }
      frame True {
        n220 = property on="多列列表框" class="MCListbox (strict)"() -> ("ItemNames"=w405:string[][], "Value"=w406:i32)  [unwired: 2 in, 2 out]
        n221 = Index Array(array=w405, index (row)=w406) -> (element=w404:string[])  [unwired: 1 in]
        n222 = Index Array(array=w404) -> (element=w403:string)  [unwired: 1 in]
        n223 = call "过滤筛选流程.vi"("字符串"=w403) -> ("匹配后偏移量"=w402:i32)  [unwired: 10 in]
        n224 = case shown="Default" w402 {
          tunnel: w403 -> [_ w407]
          frame -1 {
          }
          frame Default {
            # "步骤日志存储"
            n225 = case shown="Default" w407 {
              selector: w407 -> [w413 w415]
              tunnel: [w413 w415] -> w409
              tunnel: [string[] [] ("数组") "数组"] -> w408
              frame "读数" {
              }
              frame Default {
              }
            }
            n226 = for {
              N: 1 -> [_]
              tunnel: w409 -> [w417]
              shift-right: [w416] -> w410
              shift-left: w408 -> [w418]
              n227 = Search 1D Array(1D array=w418, element=w417) -> (index of element=w421:i32)  [unwired: 1 in]
              n228 = Format Into String(format string="%s" ("格式字符串"), w417) -> (resulting string=w422:string)  [unwired: 2 in, 1 out]
              n229 = Equal?(x=w421, y=-1) -> (x = y?=w419:bool)
              n230 = case shown="True" w419 {
                tunnel: w422 -> [_ w430]
                tunnel: w418 -> [w424 w434]
                tunnel: w417 -> [_ w433]
                tunnel: [w424 w432] -> w416
                frame False {
                }
                frame True {
                  n231 = Insert Into Array(array=w434, new element=w433) -> (w432:string[])  [unwired: 1 in]
                  n232 = case shown="\"初始化\"" w430 {
                    selector: w430 -> [w459 w462 w465]
                    tunnel: [w459 w461 w464] -> w426
                    frame Default {
                    }
                    frame "初始化" {
                      n233 = Concatenate Strings("<<" ("字符串"), w462) -> (w461:string)
                    }
                    frame "结束" {
                      n234 = Concatenate Strings(w465, ">>" ("字符串")) -> (w464:string)
                    }
                  }
                  n235 = global read "VARCODMn全局变量.vi" "状态告警区"() -> (w429:T8)
                  n236 = Unbundle By Name(w429) -> ("工作状态"=w428:u16)
                  n237 = case shown="1" w428 {
                    tunnel: [_ "【水样测试】" ("字符串") "【标样核查】" ("字符串") "【零点核查】" ("字符串") "【跨度核查】" ("字符串") "【空白测试】" ("字符串") "【平行样测试】" ("字符串") "【加标回收】" ("字符串") "【空白校准】" ("字符串") "【标样校准】" ("字符串")] -> w427
                    frame 0, Default {
                    }
                    frame 1 {
                    }
                    frame 2 {
                    }
                    frame 3 {
                    }
                    frame 4 {
                    }
                    frame 5 {
                    }
                    frame 6 {
                    }
                    frame 7 {
                    }
                    frame 8 {
                    }
                    frame 9 {
                    }
                  }
                  n238 = global read "VARCODMn全局变量.vi" "状态告警区"() -> (w449:T8)
                  n239 = Unbundle By Name(w449) -> ("id"=w448:u16)
                  n240 = global read "VARCODMn全局变量.vi" "状态告警区"() -> (w444:T8)
                  n241 = case shown="1, 21, 131" w448 {
                    tunnel: [_ "CODMn" ("table输入") "氨氮" ("table输入") "总氮" ("table输入")] -> w446
                    frame Default {
                    }
                    frame 1, 21, 131 {
                    }
                    frame 3, 92 {
                    }
                    frame 2, 76 {
                    }
                  }
                  n242 = Unbundle By Name(w444) -> ("A"=w441:sgl, "B"=w440:sgl, "K"=w439:sgl, "当前滴定数"=w438:sgl, "id"=w437:u16, "flowid"=w436:u16, "量程"=w435:u16)
                  n243 = Concatenate Strings(w427, w426) -> (w425:string)
                  n244 = Format Into String(format string="A=%#f,B=%#f,K=%#f,当前滴定数=%#f,Flow=%d-%-d-%-d" ("格式字符串"), w441, w440, w439, w438, w437, w436, w435) -> (resulting string=w442:string)  [unwired: 2 in, 1 out]
                  n245 = Get Date/Time In Seconds() -> (seconds since 1Jan1904=w445:timestamp)
                  n246 = Bundle By Name(cluster=T14 {"时间标识"=timestamp(0 s since 1904-01-01), "设备"="", "日志信息"="", "流程参数"=""} ("data in"), "时间标识"=w445, "设备"=w446, "日志信息"=w425, "流程参数"=w442) -> (w447:T14)
                  n247 = call "CODMn操作日志.vi"("data in"=w447) -> ()  [unwired: 11 in]
                }
              }
            }
            n248 = local write "数组"(w410) -> ()
          }
        }
      }
    }
    n249 = call <vilib>:"Boolean Crossing PtByPt.vi"("direction"=enum16{"either", "false-true", "true-false"}."either", "input"=w355) -> ("crossing"=w329:bool)  [unwired: 1 in]
    n250 = First Call?() -> (First Call?: T/F=w356:bool)
    n251 = Compound Arithmetic op=OR ("复合运算")(w329, w356, w313) -> (w354:bool)
    n252 = Bundle("id"=w350, "flowid"=w352, "量程"=w351) -> (w345:cluster{"id":u16, "flowid":u16, "量程":u16})  [unwired: 1 in]
    n253 = while {
      tunnel: w354 -> [w485]
      tunnel: w345 -> [w484]
      shift-right: [w481] -> _
      shift-left: _ -> [w482]
      shift-right: [w478] -> _
      shift-left: _ -> [w480]
      stop <- TRUE stop-if-true
      # "XML解析步骤显示"
      n254 = case shown="True" w485 {
        tunnel: [w487 w495] -> w478
        tunnel: [w486 w494] -> w481
        tunnel: w484 -> [_ w489]
        tunnel: w480 -> [w487 _]
        tunnel: w482 -> [w486 _]
        frame False {
        }
        frame True {
          n255 = call "斯坦道XML解析.vi"("添加的路径"="流程路径", "参数簇"=w489) -> ("步骤时间"=w490:string[], "步骤名"=w492:string[])  [unwired: 8 in]
          n256 = for {
            tunnel: w492 -> [_] mode=indexing
            tunnel: [w496] -> w493 mode=indexing
            i -> [w496]
          }
          n257 = Build Array(w492, w490) -> (w491:string[][])
          n258 = Transpose 2D Array(2D array=w491) -> (transposed array=w494:string[][])
          n259 = Number To Decimal String(number=w493) -> (decimal integer string=w495:string[])  [unwired: 1 in]
        }
      }
      n260 = Array Size(array=w478) -> (size(s)=→"总步数":i32)
      n261 = property on="多列列表框" class="MCListbox (strict)"("ItemNames"=w481, "RowHdrs[]"=w478) -> ()  [unwired: 2 in, 2 out]
    }
  }
  n262 = Obtain Queue(name (unnamed)=w6, element data type=cluster{"命令":string, "data":variant} {"命令"="", "data"=variant}) -> (queue out=w17:refnum<queue>)  [unwired: 3 in, 2 out]
  n263 = while {
    tunnel: w17 -> [w514]
    tunnel: [w508] -> _
    stop <- FALSE stop-if-true
    # "定时更新"
    n264 = control-ref of="试剂余量显示"() -> (w509:refnum<vi>)
    n265 = Get Queue Status(queue=w514) -> (queue out=w512:refnum<queue>, # elements in queue=w511:i32)  [unwired: 2 in, 6 out]
    n266 = call "最小试剂余量百分比.vi"() -> ()  [unwired: 12 in]
    n267 = case shown="0" w511 {
      tunnel: w512 -> [_ w518]
      tunnel: [_ w516] -> w508
      frame Default {
      }
      frame 0 {
        n268 = global read "CODMn断电保存全局变量.vi" "站号"() -> (w517:u16)
        n269 = Bundle By Name(cluster=cluster{"命令":string, "data":variant} {"命令"="", "data"=variant} ("元素"), "命令"="读序列号", "data"=w517) -> (w519:cluster{"命令":string, "data":variant})
        n270 = Enqueue Element(queue=w518, element=w519) -> (error out=w516:errorcluster)  [unwired: 2 in, 2 out]
      }
    }
    n271 = Wait (ms)(milliseconds to wait=u32 1000 ("等待时间（毫秒）")) -> ()  [unwired: 1 out]
    n272 = call "试剂余量展示.vi"("波形图 2"=w509) -> ("波形图"=→"试剂余量显示":sgl[][])  [unwired: 10 in]
  }
  n273 = property class="VI"(reference=w16) -> (reference out=w14:refnum<vi>, "Exec.State"=w15:T16)  [unwired: 1 in, 1 out]
  n274 = property class="VI"(reference=w13) -> (reference out=w11:refnum<vi>, "Exec.State"=w12:T16)  [unwired: 1 in, 1 out]
  n275 = case shown="\"Bad\", Default" w15 {
    tunnel: w14 -> [w522 w526]
    tunnel: [w522 w523] -> w9
    frame "Bad", Default {
    }
    frame "Idle" {
      n276 = invoke class="VI" method="Run VI"(reference=w526, "Wait until done"=FALSE ("结束前等待"), "Auto Dispose Ref"=TRUE ("自动销毁引用")) -> (reference out=w523:refnum<vi>)  [unwired: 2 in, 4 out]
    }
  }
  n277 = case shown="\"Bad\", Default" w12 {
    tunnel: w11 -> [w527 w531]
    tunnel: [w527 w528] -> w10
    frame "Bad", Default {
    }
    frame "Idle" {
      n278 = invoke class="VI" method="Run VI"(reference=w531, "Wait until done"=FALSE ("结束前等待"), "Auto Dispose Ref"=TRUE ("自动销毁引用")) -> (reference out=w528:refnum<vi>)  [unwired: 2 in, 4 out]
    }
  }
  n279 = call "设置模块队列名.vi"() -> ("Msg"=w7:string)  [unwired: 11 in]
  n280 = Obtain Notifier(name (unnamed)="CODMn" ("名称（未命名）"), notification data type=FALSE) -> (notifier out=w23:refnum<notifier>)  [unwired: 2 in, 2 out]
  n281 = Cancel Notification(0:w23) -> (8:w22:refnum<notifier>)  [unwired: 1 in, 2 out]
  n282 = Obtain Queue(name (unnamed)=w7, element data type=cluster{"命令":string, "data":variant} {"命令"="", "data"=variant}) -> (queue out=w20:refnum<queue>, error out=w31:errorcluster)  [unwired: 3 in, 1 out]
  n283 = control-ref of="测量模式下拉列表"() -> (w28:refnum<vi>)
  n284 = while {
    tunnel: w20 -> [w539]
    tunnel: w31 -> [_]
    stop <- FALSE stop-if-true
    n285 = Get Queue Status(queue=w539) -> (queue out=w535:refnum<queue>, # elements in queue=w534:i32)  [unwired: 2 in, 6 out]
    n286 = case shown="0" w534 {
      tunnel: w535 -> [_ w560]
      frame Default {
      }
      frame 0 {
        w548 = u16 0 items=["空闲"=0, "水样测试"=1, "标样核查"=2, "零点核查"=3, "跨度核查"=4, "空白测试"=5, "平行样测试"=6, "加标回收"=7, "空白校准"=8, "标样校准"=9, "初始化（清洗）"=10, "调试"=22, "填充管路"=30, "清洗管路"=31, "清洗反应杯"=32] ("工作状态")
        # "试剂填充 172 \n管路清洗108\n氨氮92\n总磷131\n总磷海水147\n总氮76\n总氮海水92"
        n287 = global read "VARCODMn全局变量.vi" "状态告警区"() -> (w550:T8)
        n288 = global read "CODMn断电保存全局变量.vi" "站号"() -> (w549:u16)
        n289 = Unbundle By Name(w550) -> ("系统时间"=w556:timestamp, "工作状态"=w547:u16)
        n290 = Bundle By Name(cluster=cluster{"命令":string, "data":variant} {"命令"="", "data"=variant} ("元素"), "命令"="读状态告警区", "data"=w549) -> (w558:cluster{"命令":string, "data":variant})
        n291 = Get Date/Time In Seconds() -> (seconds since 1Jan1904=w555:timestamp)
        n292 = Subtract(x=w555, y=w556) -> (x-y=w554:dbl)
        n293 = Equal?(x=w547, y=w548) -> (x = y?=w546:bool)
        n294 = Enqueue Element(queue=w560, element=w558) -> (queue out=w545:refnum<queue>)  [unwired: 2 in, 2 out]
        n295 = case shown="False" w546 {
          tunnel: w549 -> [w562 w570]
          tunnel: w545 -> [w563 w568]
          tunnel: [w561 w567] -> w544
          frame False {
            n296 = Bundle By Name(cluster=cluster{"命令":string, "data":variant} {"命令"="", "data"=variant} ("元素"), "命令"="读滴定曲线", "data"=w562) -> (w564:cluster{"命令":string, "data":variant})
            n297 = Enqueue Element(queue=w563, element=w564) -> (queue out=w561:refnum<queue>)  [unwired: 2 in, 2 out]
          }
          frame True {
            n298 = Bundle By Name(cluster=cluster{"命令":string, "data":variant} {"命令"="", "data"=variant} ("元素"), "命令"="读测量数据区", "data"=w570) -> (w569:cluster{"命令":string, "data":variant})
            n299 = Enqueue Element(queue=w568, element=w569) -> (queue out=w567:refnum<queue>)  [unwired: 2 in, 2 out]
          }
        }
        n300 = Absolute Value(x=w554) -> (abs(x)=w553:dbl)
        n301 = global read "VARCODMn全局变量.vi" "通讯状态"() -> (w542:bool)
        n302 = Greater Or Equal?(x=w553, y=30.0) -> (x >= y?=w551:bool)
        n303 = And(x=w551, y=w542) -> (x .and. y?=w543:bool)
        n304 = case shown="True" w543 {
          tunnel: w544 -> [_ w577]
          tunnel: w549 -> [_ w575]
          frame False {
          }
          frame True {
            n305 = Bundle By Name(cluster=T17 {"站号"=21, "量程切换"=enum."AUTO", "控制命令"=13, "模式设置"=enum."待机", "测量间隔"=0} ("参数"), "站号"=w575) -> (w573:T17)
            n306 = call "CODMn启动命令.vi"("参数"=w573) -> ("启动命令"=w576:cluster{"命令":string, "data":variant})  [unwired: 10 in]
            n307 = Enqueue Element(queue=w577, element=w576) -> ()  [unwired: 2 in, 3 out]
          }
        }
      }
    }
    n308 = Wait (ms)(milliseconds to wait=u32 1000 ("等待时间（毫秒）")) -> ()  [unwired: 1 out]
    n309 = global read "CODMn断电保存全局变量.vi" "流程路径"() -> (w538:path)
    n310 = local write "流程路径"(w538) -> ()
    n311 = global read "CODMn断电保存全局变量.vi" "MB通信方式选择"() -> (w536:enum16{"串口", "TCP"})
    n312 = global read "CODMn断电保存全局变量.vi" "远程标样校准"() -> (w533:enum16{"标液1", "标液2", "标液3", "标液4"})
    n313 = global read "CODMn断电保存全局变量.vi" "远程校准量程"() -> (w532:enum16{"低量程1", "低量程2", "高量程1", "高量程2"})
    n314 = local write "平台反控标样校准"(w533) -> ()
    n315 = local write "平台反控校准量程"(w532) -> ()
    n316 = case shown="\"TCP\"" w536 {
      tunnel: [w578 w579] -> w537
      frame "串口", Default {
        n317 = global read "CODMn断电保存全局变量.vi" "VISA Resource"() -> (w578:refnum<visa-resource-name>)
      }
      frame "TCP" {
        n318 = global read "CODMn断电保存全局变量.vi" "IP"() -> (w579:string)
      }
    }
    "字符串" <- w537
  }
  n319 = control-ref of="参数下拉列表"() -> (w29:refnum<vi>)
  n320 = control-ref of="量程下拉列表"() -> (w30:refnum<vi>)
  n321 = control-ref of="公式"() -> (w27:refnum<vi>)
  n322 = while {
    tunnel: w20 -> [w588]
    tunnel: w30 -> [w587]
    tunnel: w29 -> [w586]
    tunnel: w28 -> [w585]
    tunnel: w27 -> [w584]
    tunnel: w22 -> [w583]
    tunnel: [w582] -> _
    tunnel: w10 -> [w581]
    tunnel: w9 -> [w580]
    stop <- FALSE stop-if-true
    n323 = event shown="[3] \"流程固件\": Value Change" {
      selector: _ -> [_ _ _ _ _ _ _ _ _ _ _ _ _ _ _ _ _ _ _ _ _ _]
      dyn-events: _ -> [_ _ _ _ _ _ _ _ _ _ _ _ _ _ _ _ _ _ _ _ _ _]
      timeout: _ -> [_ _ _ _ _ _ _ _ _ _ _ _ _ _ _ _ _ _ _ _ _ _]
      tunnel: w588 -> [_ _ _ _ _ _ _ _ _ w640 _ w660 _ _ _ _ _ _ _ _ _ _]
      tunnel: w587 -> [_ _ _ _ w602 _ _ w619 _ _ _ _ _ _ _ _ _ _ _ _ _ _]
      tunnel: w586 -> [_ _ _ _ w601 _ _ w615 _ _ _ _ _ _ _ _ _ _ _ _ w735 w741]
      tunnel: w585 -> [_ _ _ _ w600 _ _ w617 _ _ _ _ _ _ _ _ _ _ _ _ _ _]
      tunnel: w584 -> [_ _ _ _ w603 _ _ w613 _ _ _ _ _ _ _ _ _ _ _ _ _ _]
      tunnel: w583 -> [_ _ _ _ _ _ _ _ _ _ _ w661 _ _ _ _ _ _ _ _ _ _]
      tunnel: [_ _ _ _ w598 _ _ _ _ _ _ _ _ _ _ _ _ _ _ _ _ _] -> w582
      tunnel: w581 -> [_ _ _ _ _ _ _ _ _ _ _ _ w668 _ _ _ _ _ _ _ _ _]
      tunnel: w580 -> [_ _ _ _ _ _ _ _ _ _ _ _ _ w672 _ _ _ _ _ _ _ _]
      event Timeout {
        n324 = event-data() -> ()  [unwired: 1 in, 3 out]
      }
      event "布尔": Value Change {
        n325 = event-data() -> ("NewVal"=w590:bool)  [unwired: 1 in, 5 out]
        n326 = case shown="False" w590 {
          frame False {
            n327 = global write "VARCODMn全局变量.vi" "权限等级"(enum16{"一级权限", "二级权限", "三级权限", "超级权限"}."一级权限" ("权限等级")) -> ()
          }
          frame True {
            n328 = global read "VARCODMn全局变量.vi" "权限密码"() -> (w594:u32[])
            n329 = global read "VARCODMn全局变量.vi" "权限等级"() -> (w593:enum16{"一级权限", "二级权限", "三级权限", "超级权限"})
            n330 = call "密码权限设置.vi"("权限输入"=w593, "权限密码"=w594) -> ("权限输出"=w592:enum16{"一级权限", "二级权限", "三级权限", "超级权限"})  [unwired: 9 in]
            n331 = global write "VARCODMn全局变量.vi" "权限等级"(w592) -> ()
          }
        }
      }
      event "权限等级": Mouse Down {
        n332 = event-data() -> ()  [unwired: 1 in, 8 out]
        n333 = global read "VARCODMn全局变量.vi" "权限密码"() -> (w597:u32[])
        n334 = global read "VARCODMn全局变量.vi" "权限等级"() -> (w596:enum16{"一级权限", "二级权限", "三级权限", "超级权限"})
        n335 = call "密码权限设置.vi"("权限输入"=w596, "权限密码"=w597) -> ("权限输出"=w595:enum16{"一级权限", "二级权限", "三级权限", "超级权限"})  [unwired: 9 in]
        n336 = global write "VARCODMn全局变量.vi" "权限等级"(w595) -> ()
      }
      event "流程固件": Value Change {
        n337 = event-data() -> ()  [unwired: 1 in, 6 out]
        n338 = call "流程固件设置对话框.vi"() -> ()  [unwired: 12 in]
      }
      event "测量模式下拉列表", "量程下拉列表", "参数下拉列表": Value Change {
        n339 = event-data() -> ()  [unwired: 1 in, 6 out]
        n340 = property class="Enum (strict)"(reference=w601) -> ("Value"=w607:enum16{"CODMn"})  [unwired: 1 in, 2 out]
        n341 = property class="Enum (strict)"(reference=w600) -> ("Value"=w604:T3)  [unwired: 1 in, 2 out]
        n342 = property class="Enum (strict)"(reference=w602) -> ("Value"=w606:enum16{"低量程1", "低量程2", "高量程1", "高量程2"})  [unwired: 1 in, 2 out]
        n343 = call "公式读取.vi"("量程"=w606, "测量模式"=w604, "测量参数"=w607) -> ("error out"=w598:errorcluster, "临界滴定数"=w599:dbl, "公式"=w605:cluster{"X^2":dbl, "X":dbl, "b":dbl})  [unwired: 6 in]
        n344 = property class="Clust (strict)"(reference=w603, "Value"=w605) -> ()  [unwired: 1 in, 2 out]
        n345 = local write "公式切换阈值滴定数(0~9999)"(w599) -> ()
      }
      event "平台反控校准量程", "平台反控标样校准": Value Change {
        n346 = event-data() -> ()  [unwired: 1 in, 6 out]
        n347 = flat-sequence {
          frame #0 {
            n348 = global write "CODMn断电保存全局变量.vi" "远程校准量程"("平台反控校准量程") -> ()
            n349 = global write "CODMn断电保存全局变量.vi" "远程标样校准"("平台反控标样校准") -> ()
          }
          frame #1 {
            n350 = call "配置文件保存.vi"() -> ()  [unwired: 12 in]
          }
        }
      }
      event "流程路径": Value Change {
        n351 = event-data() -> ()  [unwired: 1 in, 6 out]
        n352 = flat-sequence {
          frame #0 {
            n353 = local read "流程路径"() -> (w610:path)
            n354 = global write "CODMn断电保存全局变量.vi" "流程路径"(w610) -> ()
          }
          frame #1 {
            n355 = call "配置文件保存.vi"() -> ()  [unwired: 12 in]
          }
        }
      }
      event "公式单个写入": Value Change {
        n356 = event-data() -> ()  [unwired: 1 in, 6 out]
        n357 = property class="Enum (strict)"(reference=w615) -> ("Value"=w614:enum16{"CODMn"})  [unwired: 1 in, 2 out]
        n358 = property class="Enum (strict)"(reference=w617) -> ("Value"=w616:T3)  [unwired: 1 in, 2 out]
        n359 = property class="Enum (strict)"(reference=w619) -> ("Value"=w618:enum16{"低量程1", "低量程2", "高量程1", "高量程2"})  [unwired: 1 in, 2 out]
        n360 = property class="Clust (strict)"(reference=w613) -> ("Value"=w612:cluster{"X^2":dbl, "X":dbl, "b":dbl})  [unwired: 1 in, 2 out]
        n361 = call "公式写入.vi"("公式"=w612, "量程"=w618, "测量模式"=w616, "测量参数"=w614) -> ("error out"=w620:errorcluster)  [unwired: 7 in]
        n362 = case shown="No Error" w620 {
          tunnel: w616 -> [w629 _]
          tunnel: w618 -> [w627 _]
          tunnel: w612 -> [w623 _]
          tunnel: ["写入成功" ("消息") "写入失败" ("消息")] -> w611
          frame No Error {
            n363 = Equal?(x=w629, y=T3."水样测量") -> (x = y?=w626:bool)
            n364 = Equal?(x=w627, y=enum16{"低量程", "高量程"}."低量程" ("量程下拉列表")) -> (x = y?=w625:bool)
            n365 = And(x=w626, y=w625) -> (x .and. y?=w624:bool)
            n366 = case shown="True" w624 {
              tunnel: w623 -> [_ w630]
              frame False {
              }
              frame True {
                n367 = Unbundle By Name(w630) -> ("X^2"=w633:dbl, "X"=w632:dbl, "b"=w631:dbl)
                n368 = global read "CODMn断电保存全局变量.vi" "CODMn仪器参数"() -> (w634:T18)
                n369 = Bundle By Name(cluster=w634, "曲线截距"=w631, "曲线斜率"=w632, "二次多项式系数"=w633) -> (w635:T18)
                n370 = global write "CODMn断电保存全局变量.vi" "CODMn仪器参数"(w635) -> ()
              }
            }
          }
          frame Error {
          }
        }
        n371 = One Button Dialog(message=w611) -> ()  [unwired: 1 in, 1 out]
      }
      event "试剂余量设置": Value Change {
        n372 = event-data() -> ()  [unwired: 1 in, 6 out]
        n373 = call "试剂余量显示UI.vi"() -> ()  [unwired: 12 in]
      }
      event "手动启动": Value Change {
        n374 = event-data() -> ()  [unwired: 1 in, 6 out]
        n375 = call "CODMn启动参数对话框.vi"() -> ("标样浓度输出"=w638:dbl, "确认"=w637:bool, "元素"=w639:cluster{"命令":string, "data":variant})  [unwired: 9 in]
        n376 = case shown="True" w637 {
          tunnel: w640 -> [_ w650]
          tunnel: w639 -> [_ w649]
          tunnel: w638 -> [_ w642]
          frame False {
          }
          frame True {
            (unwired) u16 31 ("y")
            n377 = Enqueue Element(queue=w650, element=w649) -> ()  [unwired: 2 in, 3 out]
            n378 = global write "VARCODMn全局变量.vi" "手动启动"(TRUE ("手动启动")) -> ()
            n379 = Unbundle By Name(w649) -> ("data"=w648:variant)
            n380 = Variant To Data(type=cluster{"站号":u16, "控制命令":u16[]} {"站号"=0, "控制命令"=[]} ("输出簇"), Variant=w648) -> (data=w646:cluster{"站号":u16, "控制命令":u16[]})  [unwired: 1 in, 1 out]
            n381 = Unbundle By Name(w646) -> ("控制命令"=w645:u16[])
            n382 = Index Array(array=w645) -> (element=w644:u16)  [unwired: 1 in]
            n383 = Swap Bytes(anything=w644) -> (byte swapped=w643:u16)
            n384 = case shown="31" w643 {
              tunnel: w642 -> [_ w651 _ _ _]
              frame 0, Default {
              }
              frame 2 {
                # "标样核查"
                n385 = flat-sequence {
                  tunnel: w651 -> [w652]
                  frame #0 {
                    n386 = global read "CODMn断电保存全局变量.vi" "质控参数设置"() -> (w654:T19)
                    n387 = Bundle By Name(cluster=w654, "标准液标准浓度"=w652) -> (w653:T19)
                    n388 = global write "CODMn断电保存全局变量.vi" "质控参数设置"(w653) -> ()
                  }
                  frame #1 {
                    n389 = call "配置文件保存.vi"() -> ()  [unwired: 12 in]
                  }
                }
              }
              frame 8 {
                # "空白校准"
                n390 = property on="量程下拉列表" class="Enum (strict)"("Val(Sgnl)"=enum16{"低量程1", "低量程2", "高量程1", "高量程2"}."低量程1" ("值(信号)")) -> ()  [unwired: 2 in, 2 out]
              }
              frame 9 {
                # "标样校准"
                n391 = local read "平台反控校准量程"() -> (w656:enum16{"低量程1", "低量程2", "高量程1", "高量程2"})
                n392 = property on="量程下拉列表" class="Enum (strict)"("Val(Sgnl)"=w656) -> ()  [unwired: 2 in, 2 out]
              }
              frame 31 {
                n393 = One Button Dialog(message="“请将纯水管置于纯水中，其余管路置于清洗废液桶中”" ("消息")) -> ()  [unwired: 1 in, 1 out]
              }
            }
          }
        }
      }
      event "单步测试": Value Change {
        n394 = event-data() -> ()  [unwired: 1 in, 6 out]
        n395 = call "COMn单步调试对话框.vi"() -> ()  [unwired: 12 in]
      }
      event "停止": Value Change {
        n396 = event-data() -> ()  [unwired: 1 in, 6 out]
        n397 = Two Button Dialog(message="确认停止？" ("消息")) -> (T button?=w658:bool)  [unwired: 2 in]
        n398 = case shown="True" w658 {
          tunnel: w661 -> [_ w665]
          tunnel: w660 -> [_ w662]
          frame False {
          }
          frame True {
            n399 = Cancel Notification(0:w665) -> (8:w666:refnum<notifier>)  [unwired: 1 in, 2 out]
            n400 = Enqueue Element(queue=w662, element=cluster{"命令":string, "data":variant} {"命令"="启动", "data"=variant(cluster{"站号":u16, "控制命令":u16[]} {"站号"=21, "控制命令"=[2816]})} ("启动命令")) -> ()  [unwired: 2 in, 3 out]
            n401 = Send Notification(notification=TRUE ("通知"), notifier=w666) -> ()  [unwired: 1 in, 2 out]
          }
        }
      }
      event "设置", "参数查询": Value Change {
        n402 = event-data() -> ()  [unwired: 1 in, 6 out]
        n403 = invoke on="子面板" class="SubPnl" method="Remove VI"() -> (error out=w669:errorcluster)  [unwired: 3 in, 2 out]
        n404 = property on="窗格" class="Pane"("Origin"=T6 {"Horizontal"=0, "Vertical"=628} ("原点")) -> ()  [unwired: 2 in, 2 out]
        n405 = global write "VARCODMn全局变量.vi" "页面"(enum16{"主页", "参数页", "校准页"}."参数页" ("页面")) -> ()
        n406 = invoke on="子面板" class="SubPnl" method="Insert VI"(error in=w669, "VI Ref"=w668) -> ()  [unwired: 2 in, 4 out]
      }
      event "仪器校准": Value Change {
        n407 = event-data() -> ()  [unwired: 1 in, 6 out]
        n408 = invoke on="子面板" class="SubPnl" method="Remove VI"() -> (error out=w673:errorcluster)  [unwired: 3 in, 2 out]
        n409 = global write "VARCODMn全局变量.vi" "页面"(enum16{"主页", "参数页", "校准页"}."校准页" ("页面")) -> ()
        n410 = invoke on="子面板" class="SubPnl" method="Insert VI"(error in=w673, "VI Ref"=w672) -> ()  [unwired: 2 in, 4 out]
      }
      event "滴定曲线": Value Change {
        n411 = event-data() -> ()  [unwired: 1 in, 6 out]
        n412 = vi-ref "读取CODMn数据波形新.vi"() -> (w675:refnum<vi>)
        n413 = property class="VI"(reference=w675) -> ("Name"=w681:string)  [unwired: 1 in, 2 out]
        n414 = Open VI Reference(type specifier VI Refnum (for type only)=refnum<vi> refnum, vi path=w681, options=128 ("选项")) -> (vi reference=w679:refnum<vi>, error out=w678:errorcluster)  [unwired: 3 in]
        n415 = call-by-ref "?"(reference=w679, error in=w678) -> (reference out=w676:refnum<vi>, error out=w677:errorcluster)  [unwired: 12 in]
        n416 = Close Reference(reference=w676, error in (no error)=w677) -> ()  [unwired: 1 out]
      }
      event "历史波形", "历史波形 2": Value Change {
        n417 = event-data() -> ("CtlRef"=w683:refnum<vi>)  [unwired: 1 in, 5 out]
        n418 = property class="Bool (strict)"(reference=w683) -> ("Label.Text"=w682:string)  [unwired: 1 in, 2 out]
        n419 = call-poly <vilib>:"Read Waveforms from File.vi"() -> ("error out"=w684:errorcluster, "first waveform in record"=w685:waveform(dbl))  [unwired: 6 in, 2 out]
        n420 = case shown="No Error" w684 {
          tunnel: w685 -> [w689 _]
          tunnel: w682 -> [w686 _]
          frame No Error {
            n421 = Unbundle By Name(w689) -> ("t0"=w688:timestamp, "Y"=w687:dbl[])  [unwired: 2 out]
            n422 = case shown="\"历史波形\", Default" w686 {
              tunnel: w688 -> [w690 w693]
              tunnel: w687 -> [w691 w692]
              frame "历史波形2" {
                n423 = global write "VARCODMn全局变量.vi" "温度波形时间"(w690) -> ()
                n424 = global write "VARCODMn全局变量.vi" "温度曲线"(w691) -> ()
                n425 = global write "VARCODMn全局变量.vi" "时间-温度"(w691) -> ()
              }
              frame "历史波形", Default {
                n426 = global write "VARCODMn全局变量.vi" "波形时间"(w693) -> ()
                n427 = global write "VARCODMn全局变量.vi" "ORP滴定曲线"(w692) -> ()
                n428 = global write "VARCODMn全局变量.vi" "滴定数-ORP值"(w692) -> ()
              }
            }
          }
          frame Error {
            n429 = One Button Dialog(message="打开失败" ("消息")) -> ()  [unwired: 1 in, 1 out]
          }
        }
      }
      event "返回", "返回 2", "返回 3": Value Change {
        n430 = event-data() -> ()  [unwired: 1 in, 6 out]
        n431 = global write "VARCODMn全局变量.vi" "页面"(enum16{"主页", "参数页", "校准页"}."主页" ("页面")) -> ()
        n432 = property on="窗格" class="Pane"("Origin"=T6 {"Horizontal"=0, "Vertical"=0} ("原点")) -> ()  [unwired: 2 in, 2 out]
      }
      event "公式.X^2", "公式.X", "公式.b", "公式切换阈值滴定数(0~9999)": Mouse Down {
        n433 = event-data() -> ("CtlRef"=w700:refnum<vi>)  [unwired: 1 in, 5 out]
        n434 = property class="DigNum (strict)"(reference=w700) -> (reference out=w698:refnum<vi>, "Value"=w699:dbl)  [unwired: 1 in, 1 out]
        n435 = call "数字键盘.vi"("OldNumber"=w699) -> ("NewNumber"=w697:dbl)
        n436 = property class="DigNum (strict)"(reference=w698, "Val(Sgnl)"=w697) -> ()  [unwired: 1 in, 2 out]
      }
      event "读公式": Value Change {
        n437 = event-data() -> ()  [unwired: 1 in, 6 out]
      }
      event "写公式": Value Change {
        n438 = event-data() -> ()  [unwired: 1 in, 6 out]
        n439 = Two Button Dialog(message="即将将左侧拟合公式写入仪器所有模式\n请选择是否写入?" ("消息"), 1:"否" ("F按钮名称（“取消”）"), 2:"是" ("T按钮名称（“确定”）")) -> (T button?=w701:bool)
        n440 = case shown="True" w701 {
          frame False {
          }
          frame True {
            n441 = for {
              N: 7 -> [_]
              shift-right: [w710] -> _
              shift-left: T3."水样测量" ("测量模式下拉列表") -> [w711]
              tunnel: [w709] -> w705
              n442 = call "公式写入.vi"("临界滴定数"="公式切换阈值滴定数(0~9999)", "公式"="公式", "量程"="量程下拉列表", "测量模式"=w711, "测量参数"="参数下拉列表") -> ("error out"=w715:errorcluster)  [unwired: 6 in]
              n443 = Increment(x=w711) -> (x+1=w710:T3)
              n444 = case shown="No Error" w715 {
                tunnel: w711 -> [w724 _]
                tunnel: "量程下拉列表" -> [w723 _]
                tunnel: "公式" -> [w719 _]
                tunnel: ["写入成功" ("消息") "写入失败" ("消息")] -> w709
                frame No Error {
                  n445 = Equal?(x=w724, y=T3."水样测量") -> (x = y?=w722:bool)
                  n446 = Equal?(x=w723, y=enum16{"低量程1", "低量程2", "高量程1", "高量程2"}."低量程1") -> (x = y?=w721:bool)
                  n447 = And(x=w722, y=w721) -> (x .and. y?=w720:bool)
                  n448 = case shown="True" w720 {
                    tunnel: w719 -> [_ w725]
                    frame False {
                    }
                    frame True {
                      n449 = Unbundle By Name(w725) -> ("X^2"=w728:dbl, "X"=w727:dbl, "b"=w726:dbl)
                      n450 = global read "CODMn断电保存全局变量.vi" "CODMn仪器参数"() -> (w729:T18)
                      n451 = Bundle By Name(cluster=w729, "曲线截距"=w726, "曲线斜率"=w727, "二次多项式系数"=w728) -> (w730:T18)
                      n452 = global write "CODMn断电保存全局变量.vi" "CODMn仪器参数"(w730) -> ()
                    }
                  }
                }
                frame Error {
                }
              }
            }
            n453 = One Button Dialog(message=w705) -> ()  [unwired: 1 in, 1 out]
          }
        }
      }
      event "量程切换阈值读取": Value Change {
        n454 = event-data() -> ()  [unwired: 1 in, 6 out]
        n455 = property class="Enum (strict)"(reference=w735) -> ("Value"=w734:enum16{"CODMn"})  [unwired: 1 in, 2 out]
        n456 = call "量程读取.vi"("测量参数"=w734) -> ("error out"=w732:errorcluster)  [unwired: 9 in, 1 out]
        n457 = case shown="Error" w732 {
          tunnel: ["读取成功" ("消息") "读取失败" ("消息")] -> w733
          frame No Error {
          }
          frame Error {
          }
        }
        n458 = One Button Dialog(message=w733) -> ()  [unwired: 1 in, 1 out]
      }
      event "量程切换阈值写入": Value Change {
        n459 = event-data() -> ()  [unwired: 1 in, 6 out]
        n460 = property class="Enum (strict)"(reference=w741) -> ("Value"=w740:enum16{"CODMn"})  [unwired: 1 in, 2 out]
        n461 = call "量程写入.vi"("测量参数"=w740) -> ("error out"=w738:errorcluster)  [unwired: 9 in]
        n462 = case shown="No Error" w738 {
          tunnel: ["写入成功" ("消息") "写入失败" ("消息")] -> w739
          frame No Error {
          }
          frame Error {
          }
        }
        n463 = One Button Dialog(message=w739) -> ()  [unwired: 1 in, 1 out]
      }
    }
  }
  n464 = call "Close TimingControl.vi"("error in (no error)"=w1, "TimingControl in"=w2) -> ()  [unwired: 9 in, 1 out]
